vi "MAC_16-5.vi"(9 "b":fxp<+/-,16,5>, 10 "sclr":bool, 11 "a":fxp<+/-,16,5>) -> (3 "s":fxp<+/-,32,10>)   [LabVIEW 2019]
uses:
  <vilib>/rvi/IPIntegrationNode/IPINode_Typedef/niFpgaIPINodeSupportedFamilies.ctl
  <vilib>/rvi/IPIntegrationNode/IPINode_Utilities/niFpgaIPINodeSimCore.vi
  <vilib>/rvi/XilinxIP/XIPIN_XNode/niFpgaXIPIN.xnode
  hysteresis_fxp_16_5/MAC01/Multiply_Accumulator_ED2DB7673BE24B9DA25B94993391B6B2.dll
  <vilib>/rvi/IPIntegrationNode/IPINode_Xnode/niFpgaIPINode.xnode
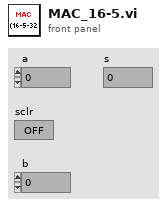
[diagram p1: front panel]
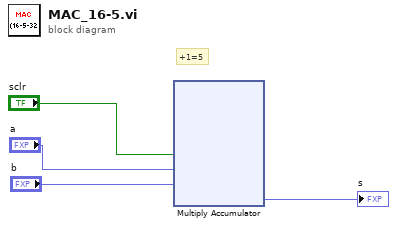
[diagram p0: block diagram]
diagram:
  # "+1=5"
  n1 = xnode ("Multiply Accumulator")("sclr"="sclr", "a"="a", "b"="b") -> ("s"=→"s":fxp<+/-,32,10>)  [unwired: 2 in]
